vi "readBuffer.vi"(8 "error in (no error)":errorcluster, 11 "Electrometer in":refnum<class "Electrometer.lvclass">) -> (0 "error out":errorcluster, 2 "data":string, 3 "Electrometer out":refnum<class "Electrometer.lvclass">)   [LabVIEW 2016, in "Electrometer.lvclass"]
uses:
  Electrometer.lvclass
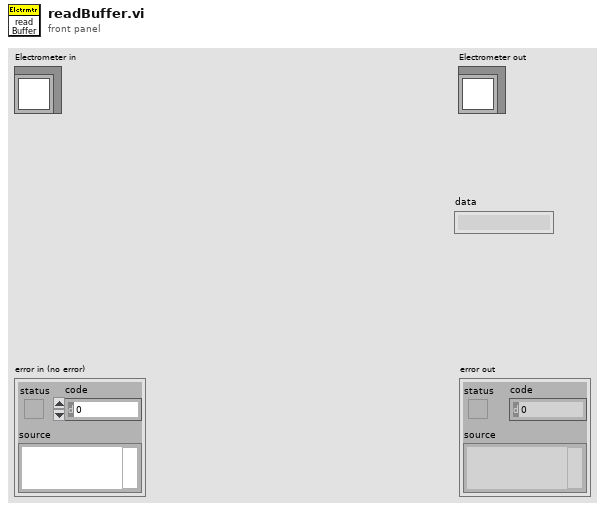
[diagram p1: front panel]
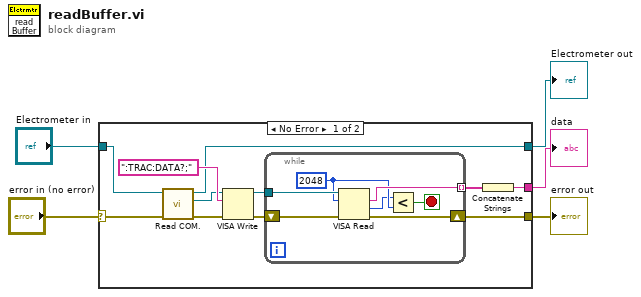
[diagram p0: block diagram]
diagram:
  n1 = case shown="No Error" "error in (no error)" {
    selector: "error in (no error)" -> [w13 w25]
    tunnel: [w11 w25] -> w4
    tunnel: [w12 w24] -> w2
    tunnel: "Electrometer in" -> [w15 w24]
    tunnel: [w7 _] -> w1
    frame No Error {
      n2 = call "Read COM..vi"("error in (no error)"=w13, "Electrometer in"=w15) -> ("error out"=w8:errorcluster, "VISA"=w14:refnum<visa-resource-name>, "Electrometer out"=w12:refnum<class "Electrometer.lvclass">)  [unwired: 7 in]
      n3 = VISA Write(VISA resource name=w14, write buffer=":TRAC:DATA?;", error in (no error)=w8) -> (VISA resource name out=w10:refnum<visa-resource-name>, error out=w9:errorcluster)  [unwired: 1 out]
      n4 = while {
        tunnel: [w23] -> w6 mode=indexing
        tunnel: w10 -> [w20]
        shift-right: [w22] -> w11
        shift-left: w9 -> [w21]
        stop <- w18 stop-if-true
        w19 = u32 2048 ("byte count")
        n5 = VISA Read(VISA resource name=w20, byte count=w19, error in (no error)=w21) -> (read buffer=w23:string, return count=w17:u32, error out=w22:errorcluster)  [unwired: 1 out]
        n6 = Less?(x=w17, y=w19) -> (x < y?=w18:bool)
      }
      n7 = Concatenate Strings(w6) -> (w7:string)
    }
    frame Error {
    }
  }
  "error out" <- w4
  "Electrometer out" <- w2
  "data" <- w1
